vi "Add Weighted Images.vi"   [LabVIEW 2020, in "image.lvlib"]
doc: "Combine two images A and B scaled by their corresponding scaling factors - with the addition of an optional constant. Pixel values will saturate at their maximum values."
uses:
  image.lvlib
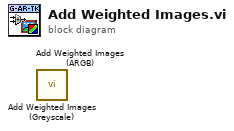
[diagram p0: block diagram]
diagram:
  n1 = call "Add Weighted Images (Greyscale).vi"() -> ()  [unwired: 10 in, 2 out]
  n2 = call "Add Weighted Images (ARGB).vi"() -> ()  [unwired: 10 in, 2 out]
